vi "IO@InitIOPort__Parameter.vi"(1 "ParamterIn":string) -> (0 "ParamterOut":string)   [LabVIEW 2020]
panel:
  in  "IOSelect":string(combo)
  in  "Confirm":bool
  # "IO@InitPort $IOCard"
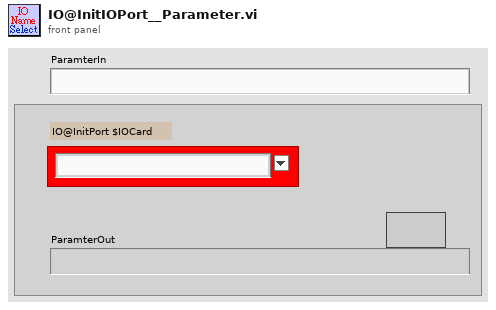
[diagram p1: front panel]
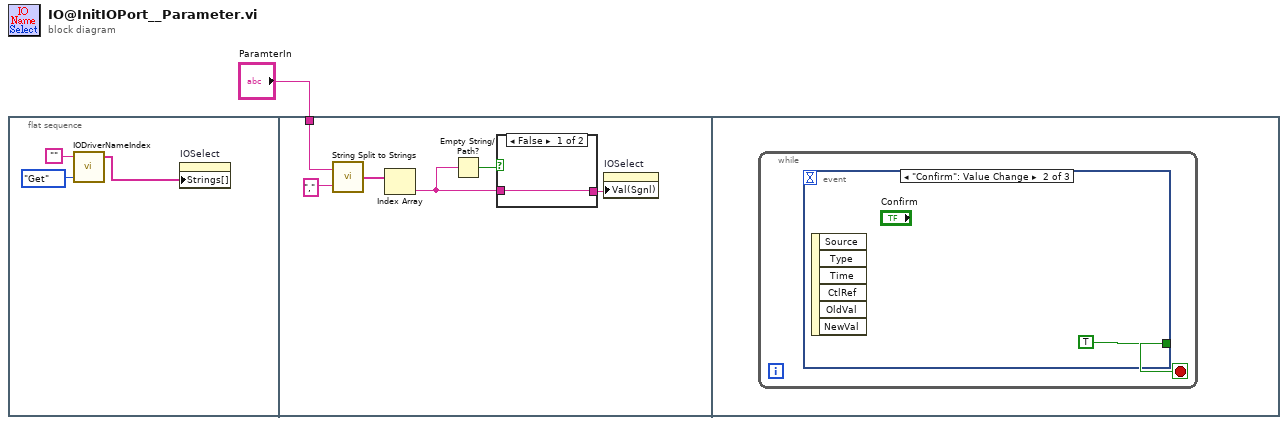
[diagram p0: block diagram]
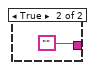
[diagram p2: hidden frame]
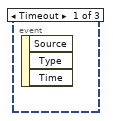
[diagram p3: hidden frame]
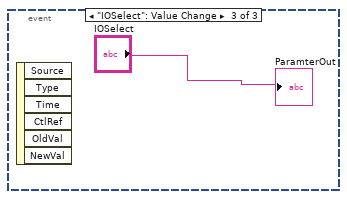
[diagram p4: hidden frame]
diagram:
  n1 = flat-sequence {
    tunnel: "ParamterIn" -> [w8]
    frame #0 {
      n2 = call "IODriverNameIndex.vi"("OP"=enum16{"Get", "Update", "Init"}."Get", "IODriverName"="") -> ("IODriverList"=w2:string[])  [unwired: 1 in, 2 out]
      n3 = property on="IOSelect" class="CmbBox"("Strings[]"=w2) -> ()  [unwired: 2 in, 2 out]
    }
    frame #1 {
      n4 = call "String Split to Strings.vi"("search string/char (-)"=",", "String"=w8) -> ("Array"=w9:string[])
      n5 = Index Array(array=w9) -> (element=w6:string)  [unwired: 1 in]
      n6 = Empty String/Path?(string/path=w6) -> (empty?=w7:bool)
      n7 = case shown="False" w7 {
        tunnel: w6 -> [w11 _]
        tunnel: [w11 ""] -> w5
        frame False {
        }
        frame True {
        }
      }
      n8 = property on="IOSelect" class="CmbBox"("Val(Sgnl)"=w5) -> ()  [unwired: 2 in, 2 out]
    }
    frame #2 {
      n9 = while {
        stop <- w13 stop-if-true
        n10 = event shown="[1] \"Confirm\": Value Change" {
          selector: _ -> [_ _ _]
          dyn-events: _ -> [_ _ _]
          timeout: _ -> [_ _ _]
          tunnel: [_ TRUE _] -> w13
          event Timeout {
            n11 = event-data() -> ()  [unwired: 1 in, 3 out]
          }
          event "Confirm": Value Change {
            n12 = event-data() -> ()  [unwired: 1 in, 6 out]
          }
          event "IOSelect": Value Change {
            n13 = event-data() -> ()  [unwired: 1 in, 6 out]
            "ParamterOut" <- "IOSelect"
          }
        }
      }
    }
  }
